vi "FlatToRichcif_template_Result.vi"(5 "OutputClusterType":T1, 11 "InputCluster":T2) -> (3 "OutputCluster":T1)   [LabVIEW 2021, in "Template_server.lvlib"]
uses:
  Template_server.lvlib
  cif_template_Result_Flat.ctl
  cif_template_Result.ctl
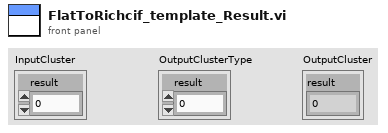
[diagram p1: front panel]
types:
  T1 = typedef "Template_server.lvlib/cif_template_Result.ctl" = cluster{"result":i32}
  T2 = typedef "Template_server.lvlib/cif_template_Result_Flat.ctl" = cluster{"result":i32}
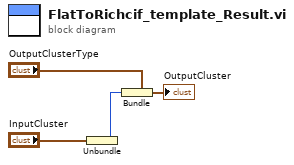
[diagram p0: block diagram]
diagram:
  n1 = Unbundle "Unbundle"("InputCluster") -> ("result"=w1:i32)
  n2 = Bundle "Bundle"(cluster="OutputClusterType", "result"=w1) -> (→"OutputCluster":T1)
